vi "Gaus Function.vi"(10 "Fit params":T1={"Amplitude"=1000.0, "Center"=694.3, "Width"=0.4}, 11 "X":dbl[](array[numeric])) -> (3 "Y":dbl[](array[numeric]))   [LabVIEW 2016]
uses:
  Peak Parameters.ctl
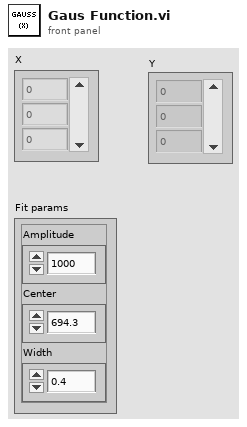
[diagram p1: front panel]
types:
  T1 = typedef "Peak Parameters.ctl" = cluster{"Amplitude":dbl, "Center":dbl, "Width":dbl}
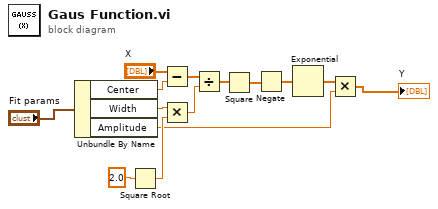
[diagram p0: block diagram]
diagram:
  n1 = Unbundle By Name("Fit params") -> ("Center"=w13:dbl, "Width"=w11:dbl, "Amplitude"=w2:dbl)
  n2 = Square Root(x=2.0 ("y")) -> (sqrt(x)=w8:dbl)
  n3 = Subtract(x="X", y=w13) -> (x-y=w9:dbl[])
  n4 = Multiply(x=w11, y=w8) -> (x*y=w7:dbl)
  n5 = Divide(x=w9, y=w7) -> (x/y=w6:dbl[])
  n6 = Square(x=w6) -> (x^2=w5:dbl[])
  n7 = Negate(x=w5) -> (-x=w4:dbl[])
  n8 = Exponential(1:w4) -> (0:w3:dbl[])
  n9 = Multiply(x=w3, y=w2) -> (x*y=→"Y":dbl[])
